vi "midiOutOpen.vi"(8 "error in":errorcluster, 10 "DeviceID":u32, 11 "midi in":refnum<class "midi.lvclass">) -> (0 "error out":errorcluster, 2 "phmo":u32, 3 "midi out":refnum<class "midi.lvclass">)   [LabVIEW 2020, in "midi.lvclass"]
uses:
  midi.lvclass
  midi.lvclass/midi.ctl
  winmm.dll
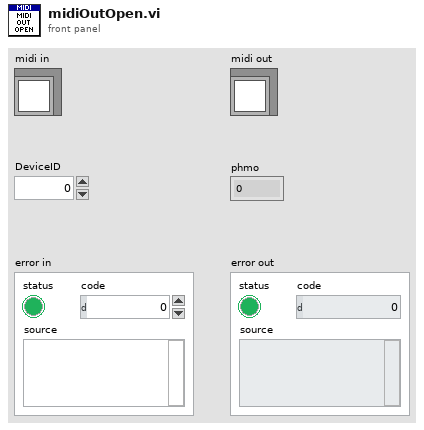
[diagram p1: front panel]
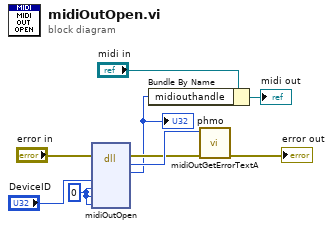
[diagram p0: block diagram]
diagram:
  w9 = 0
  n1 = dll-call lib="winmm.dll" fn="midiOutOpen"(error in="error in", "uDeviceID"="DeviceID", "dwCallback"=w9, "dwInstance"=w9, "fdwOpen"=w9) -> (error out=w7:errorcluster, "errorcode"=w8:i32, "phmo"=w3:u32)  [unwired: 7 in, 1 out]
  "phmo" <- w3
  n2 = Bundle By Name(cluster="midi in", "midiouthandle"=w3) -> (→"midi out":refnum<class "midi.lvclass">)
  n3 = call "midiOutGetErrorTextA.vi"("error in"=w7, "Error Code"=w8) -> ("error out"=→"error out":errorcluster)  [unwired: 9 in]
